vi "InStepType.vi"(11 "Label":string) -> (3 "Numeric":i32)   [LabVIEW 2010]
panel:
  out "String":string
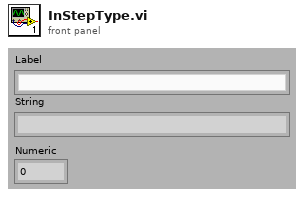
[diagram p1: front panel]
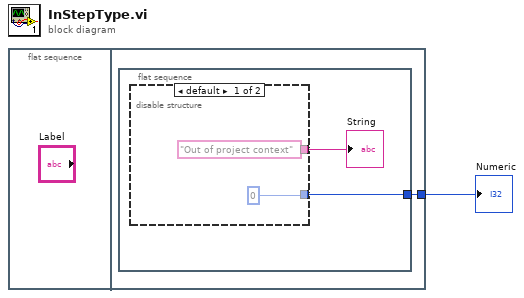
[diagram p0: block diagram]
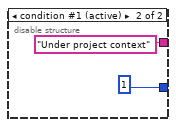
[diagram p2: hidden frame]
diagram:
  n1 = flat-sequence {
    tunnel: [w2] -> w1
    frame #0 {
    }
    frame #1 {
      n2 = flat-sequence {
        tunnel: [w3] -> w2
        frame #0 {
          n3 = disable-structure shown="default" {
            disable-tunnel: ["Out of project context" ("String") "Under project context" ("String")] -> w4
            disable-tunnel: [0 ("Numeric") 1 ("Numeric")] -> w3
            frame condition #0 {
            }
            frame condition #1 (active) {
            }
          }
          "String" <- w4
        }
      }
    }
  }
  "Numeric" <- w1
